vi "Emballage_BDD_messageHorsConnection.vi"(8 "Error in":errorcluster caption="Error in (no error)") -> (0 "Error out":errorcluster, 3 "Quitter":bool)   [LabVIEW 2017]
panel:
  in  "btn_continuer":bool
  in  "Bouton Arrêt du processus":bool
  out "Titre":string
  out "Détail":string
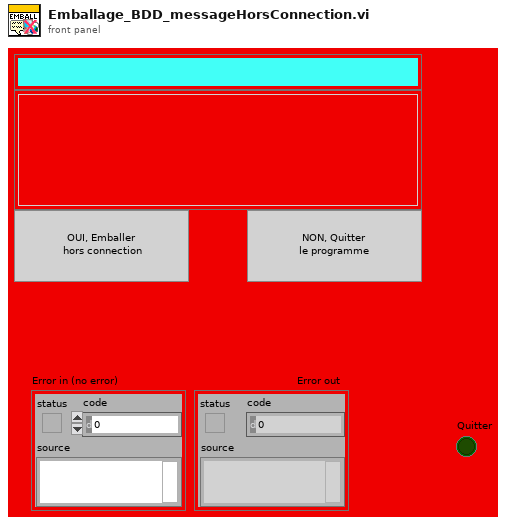
[diagram p1: front panel]
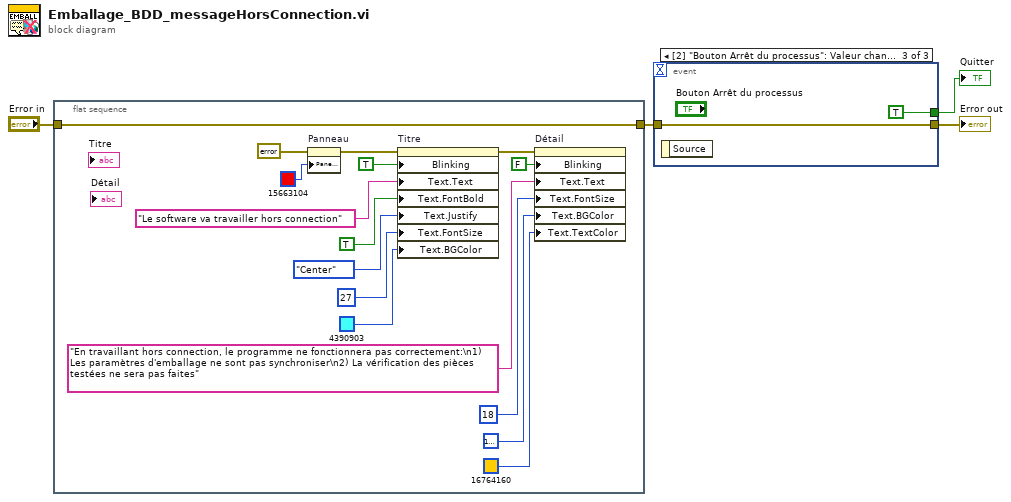
[diagram p0: block diagram]
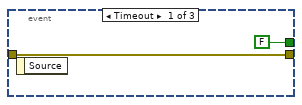
[diagram p2: hidden frame]
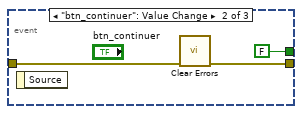
[diagram p3: hidden frame]
diagram:
  n1 = flat-sequence {
    tunnel: [w20] -> w1
    tunnel: "Error in" -> [w20]
    frame #0 {
      n2 = property on="Panneau" class="Pann"(error in=errorcluster {"status"=FALSE, "code"=0, "source"=""} ("entrée d'erreur (pas d'erreur)"), "PaneColor"=u32 15663104) -> (error out=w13:errorcluster)  [unwired: 1 in, 1 out]
      n3 = property on="Titre" class="Ch"(error in=w13, "Blinking"=TRUE ("Clignotant"), "Text.Text"="Le software va travailler hors connection" ("Titre"), "Text.FontBold"=TRUE ("Texte.Police:Gras"), "Text.Justify"=enum16{"Left", "Center", "Right"}."Center" ("Texte.Justification"), "Text.FontSize"=u32 27 ("Texte.Police:Taille"), "Text.BGColor"=u32 4390903) -> (error out=w9:errorcluster)  [unwired: 1 in, 1 out]
      n4 = property on="Détail" class="Ch"(error in=w9, "Blinking"=FALSE ("Clignotant"), "Text.Text"="En travaillant hors connection, le programme ne fonctionnera pas correctement:\n1) Les paramètres d'emballage ne sont pas synchroniser\n2) La vérification des pièces testées ne sera pas faites" ("Détail"), "Text.FontSize"=u32 18 ("Texte.Police:Taille"), "Text.BGColor"=u32 16777216, "Text.TextColor"=u32 16764160) -> ()  [unwired: 1 in, 2 out]
    }
  }
  n5 = event shown="[2] \"Bouton Arrêt du processus\": Valeur changée" {
    selector: _ -> [_ _ _]
    dyn-events: _ -> [_ _ _]
    timeout: _ -> [_ _ _]
    tunnel: [w22 w24 w27] -> w4
    tunnel: w1 -> [w22 w25 w27]
    tunnel: [FALSE FALSE TRUE] -> w3
    event Timeout {
      n6 = event-data() -> ()  [unwired: 1 in, 1 out]
    }
    event "btn_continuer": Value Change {
      n7 = event-data() -> ()  [unwired: 1 in, 1 out]
      n8 = call <vilib>:"Clear Errors.vi"("error in (no error)"=w25) -> ("error out"=w24:errorcluster)  [unwired: 5 in, 1 out]
    }
    event "Bouton Arrêt du processus": Value Change {
      n9 = event-data() -> ()  [unwired: 1 in, 1 out]
    }
  }
  "Error out" <- w4
  "Quitter" <- w3
